vi "Example_AOU_AWG_Array.vi"() -> ()   [LabVIEW 2013]
panel:
  out "Points >=30":bool[](array[boolean])
  out "Points":i32[](array[numeric])
  in  "AWG":u32
  in  "Run":bool
  in  "waveformData":dbl[][](array[numeric]) min=-1.0 max=1.0 step=0.01
  in  "waveformType":i32(ring) items=["Analog"=0, "IQ"=2, "IQ (polar)"=3]
  out "errorOut":errorcluster
  in  "Close":bool
  in  "Prescaler":u32
  in  "Cycles":u32
  in  "Start Delay":u32
  in  "Trigger Mode":T1(ring)
  in  "nSlot":i32=7
  in  "nChassis":i32=1
  in  "partNumber":string="SD-PXE-AOU-H0002-128"
  # "AWG Data"
  # "Module Under Test"
  # "AWG Parameters"
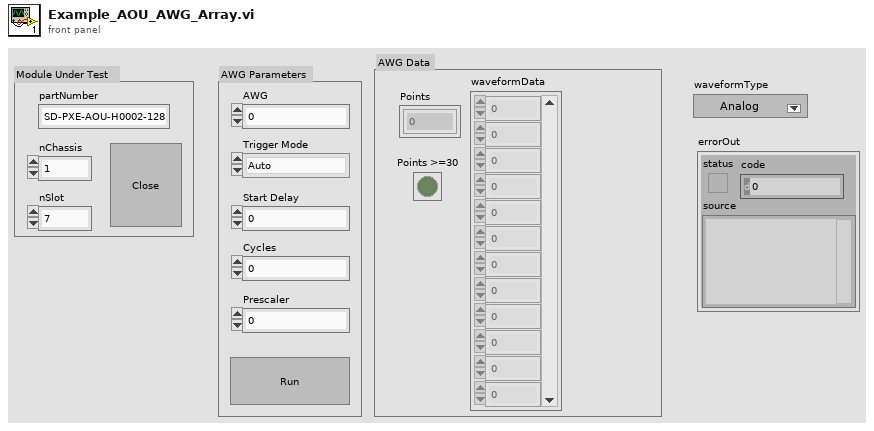
[diagram p1: front panel]
types:
  T1 = enum32{"Auto", "VI/HVI Trigger", "External Trigger"}
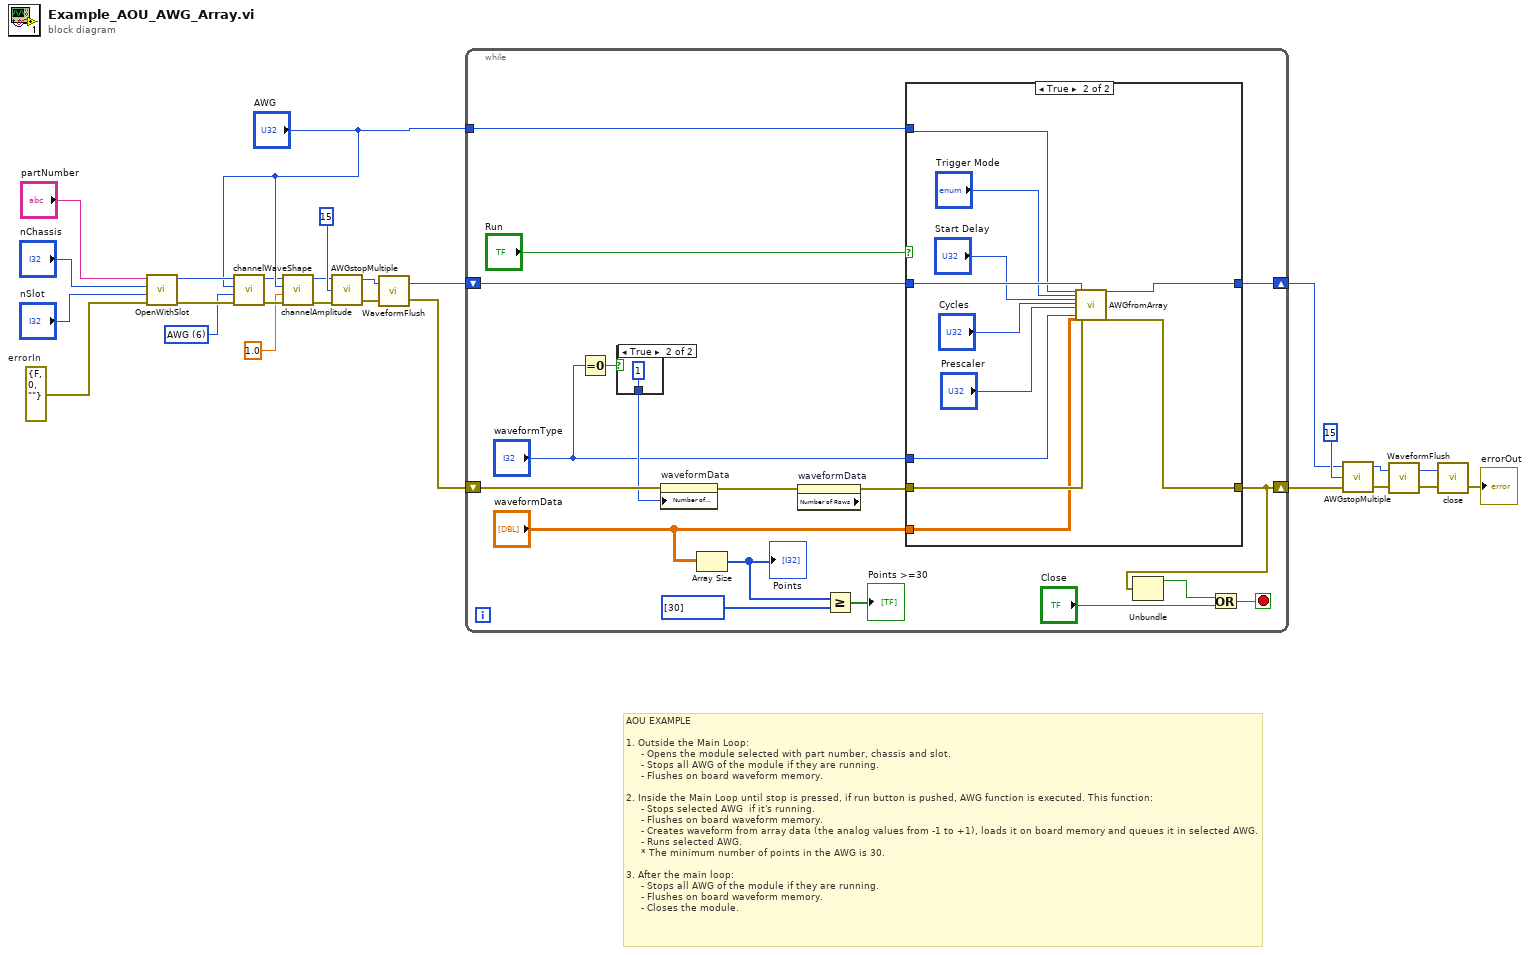
[diagram p0: block diagram]
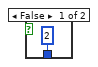
[diagram p2: hidden frame]
diagram:
  w7 = 6 items=["None"=-1, "Sinusoidal"=1, "Triangular"=2, "Sawtooth"=3, "Square"=4, "DC"=5, "AWG"=6] ("waveShape")
  w11 = errorcluster {"status"=FALSE, "code"=0, "source"=""}  # errorIn
  # "AOU EXAMPLE\n\n1. Outside the Main Loop:\n     - Opens the module selected with part number, chassis and slot.\n     - Stops all AWG of the module if they are running.\n     - Flushes on board waveform memory.\n\n2. Inside the Main Loop until stop is pressed, if run button is pushed, AWG function is executed. This function:\n     - Stops selected AWG  if it's running.\n     - Flushes on board waveform memory.\n     - Creates waveform from array data (the analog values from -1 to +1), loads it on board memory and queues it in selected AWG.\n     - Runs selected AWG.\n     * The minimum number of points in the AWG is 30.  \n\n3. After the main loop:\n     - Stops all AWG of the module if they are running.\n     - Flushes on board waveform memory.\n     - Closes the module."
  n1 = call <vilib>:"OpenWithSlot.vi"("errorIn"=w11, "nSlot"="nSlot", "nChassis"="nChassis", "partNumber"="partNumber") -> ("errorOut"=w8:errorcluster, "moduleID"=w9:i32)  [unwired: 2 in]
  n2 = call <vilib>:"channelWaveShape.vi"("errorIn"=w8, "waveShape"=w7, "nChannel"="AWG", "moduleID"=w9) -> ("errorOut"=w6:errorcluster, "moduleIDOut"=w3:i32)  [unwired: 2 in]
  n3 = call <vilib>:"channelAmplitude.vi"("errorIn"=w6, "amplitude"=1.0, "nChannel"="AWG", "moduleID"=w3) -> ("errorOut"=w5:errorcluster, "moduleIDOut"=w2:i32)  [unwired: 2 in]
  n4 = call <vilib>:"AWGstopMultiple.vi"("errorIn"=w5, "AWGmask"=15, "moduleID"=w2) -> ("errorOut"=w14:errorcluster, "moduleIDOut"=w13:i32)  [unwired: 1 in]
  n5 = call <vilib>:"WaveformFlush.vi"("errorIn"=w14, "moduleID"=w13) -> ("errorOut"=w23:errorcluster, "moduleIDOut"=w24:i32)
  n6 = while {
    shift-right: [w38] -> w18
    shift-left: w23 -> [w37]
    shift-right: [w42] -> w10
    shift-left: w24 -> [w44]
    tunnel: "AWG" -> [w31]
    stop <- w41 stop-if-true
    n7 = Equal To 0?(x="waveformType") -> (x = 0?=w35:bool)
    n8 = case shown="True" w35 {
      tunnel: [2 1] -> w36
      frame False {
      }
      frame True {
      }
    }
    n9 = property on="waveformData" class="Arr (strict)"(error in=w37, "Number of Columns"=w36) -> (error out=w32:errorcluster)  [unwired: 1 in, 1 out]
    n10 = Array Size(array="waveformData") -> (size(s)=w29:i32[])
    "Points" <- w29
    n11 = property on="waveformData" class="Arr (strict)" props=["Number of Rows"](error in=w32) -> (error out=w33:errorcluster)  [unwired: 1 in, 2 out]
    n12 = Greater Or Equal?(x=w29, y=i32[] [30]) -> (x >= y?=→"Points >=30":bool[])
    n13 = case shown="True" "Run" {
      tunnel: w44 -> [w48 w59]
      tunnel: w33 -> [w47 w54]
      tunnel: [w47 w53] -> w38
      tunnel: [w48 w52] -> w42
      tunnel: "waveformData" -> [_ w51]
      tunnel: "waveformType" -> [_ w50]
      tunnel: w31 -> [_ w49]
      frame False {
      }
      frame True {
        n14 = call <vilib>:"AWGfromArray.vi"("nAWG"=w49, "triggerMode"="Trigger Mode", "startDelay"="Start Delay", "cycles"="Cycles", "prescaler"="Prescaler", "waveformType"=w50, "waveformData"=w51, "moduleID"=w59, "errorIn"=w54) -> ("moduleIDOut"=w52:i32, "errorOut"=w53:errorcluster)  [unwired: 17 in]
      }
    }
    n15 = Unbundle(w38) -> ("status"=w40:bool)  [unwired: 2 out]
    n16 = Or(x=w40, y="Close") -> (x .or. y?=w41:bool)
  }
  n17 = call <vilib>:"AWGstopMultiple.vi"("errorIn"=w18, "AWGmask"=15, "moduleID"=w10) -> ("errorOut"=w17:errorcluster, "moduleIDOut"=w16:i32)  [unwired: 1 in]
  n18 = call <vilib>:"WaveformFlush.vi"("errorIn"=w17, "moduleID"=w16) -> ("errorOut"=w21:errorcluster, "moduleIDOut"=w20:i32)
  n19 = call <vilib>:"close.vi"("errorIn"=w21, "moduleID"=w20) -> ("errorOut"=→"errorOut":errorcluster)  [unwired: 1 in]
